vi "Unflatten-EventType.vi"(8 "error in (no error)":errorcluster, 11 "Event Binary Data In":string) -> (0 "error out":errorcluster, 3 "EventType":T1=enum."SDL_EVENT_QUIT")   [LabVIEW 2026, in "SDL3.lvlib" / "Events.lvlib"]
uses:
  Events.lvlib
  EventType--enum.ctl
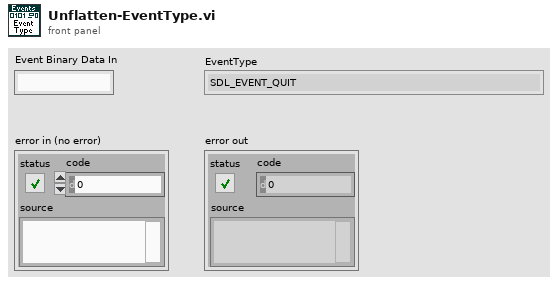
[diagram p1: front panel]
types:
  T1 = typedef "SDL3.lvlib/Events.lvlib/EventType--enum.ctl" = enum16{"LV_NONE", "LV_UNSUPPORTED", "SDL_EVENT_QUIT", "SDL_EVENT_LOCALE_CHANGED", "SDL_EVENT_SYSTEM_THEME_CHANGED", "SDL_EVENT_DISPLAY_ORIENTATION", "SDL_EVENT_DISPLAY_ADDED", "SDL_EVENT_DISPLAY_REMOVED", "SDL_EVENT_DISPLAY_MOVED", "SDL_EVENT_DISPLAY_DESKTOP_MODE_CHANGED", "SDL_EVENT_DISPLAY_CURRENT_MODE_CHANGED", "SDL_EVENT_DISPLAY_CONTENT_SCALE_CHANGED", "SDL_EVENT_WINDOW_SHOWN", "SDL_EVENT_WINDOW_HIDDEN", "SDL_EVENT_WINDOW_EXPOSED", "SDL_EVENT_WINDOW_MOVED", "SDL_EVENT_WINDOW_RESIZED", "SDL_EVENT_WINDOW_PIXEL_SIZE_CHANGED", "SDL_EVENT_WINDOW_METAL_VIEW_RESIZED", "SDL_EVENT_WINDOW_MINIMIZED", "SDL_EVENT_WINDOW_MAXIMIZED", "SDL_EVENT_WINDOW_RESTORED", "SDL_EVENT_WINDOW_MOUSE_ENTER", "SDL_EVENT_WINDOW_MOUSE_LEAVE", "SDL_EVENT_WINDOW_FOCUS_GAINED", "SDL_EVENT_WINDOW_FOCUS_LOST", "SDL_EVENT_WINDOW_CLOSE_REQUESTED", "SDL_EVENT_WINDOW_HIT_TEST", "SDL_EVENT_WINDOW_ICCPROF_CHANGED", "SDL_EVENT_WINDOW_DISPLAY_CHANGED", "SDL_EVENT_WINDOW_DISPLAY_SCALE_CHANGED", "SDL_EVENT_WINDOW_SAFE_AREA_CHANGED", "SDL_EVENT_WINDOW_OCCLUDED", "SDL_EVENT_WINDOW_ENTER_FULLSCREEN", "SDL_EVENT_WINDOW_LEAVE_FULLSCREEN", "SDL_EVENT_WINDOW_DESTROYED", "SDL_EVENT_WINDOW_HDR_STATE_CHANGED", "SDL_EVENT_KEY_DOWN", "SDL_EVENT_KEY_UP", "SDL_EVENT_TEXT_EDITING", "SDL_EVENT_TEXT_INPUT", "SDL_EVENT_KEYMAP_CHANGED", "SDL_EVENT_KEYBOARD_ADDED", "SDL_EVENT_KEYBOARD_REMOVED", "SDL_EVENT_TEXT_EDITING_CANDIDATES", "SDL_EVENT_MOUSE_MOTION", "SDL_EVENT_MOUSE_BUTTON_DOWN", "SDL_EVENT_MOUSE_BUTTON_UP", "SDL_EVENT_MOUSE_WHEEL", "SDL_EVENT_MOUSE_ADDED", "SDL_EVENT_MOUSE_REMOVED", "SDL_EVENT_JOYSTICK_AXIS_MOTION", "SDL_EVENT_JOYSTICK_BALL_MOTION", "SDL_EVENT_JOYSTICK_HAT_MOTION", "SDL_EVENT_JOYSTICK_BUTTON_DOWN", "SDL_EVENT_JOYSTICK_BUTTON_UP", "SDL_EVENT_JOYSTICK_ADDED", "SDL_EVENT_JOYSTICK_REMOVED", "SDL_EVENT_JOYSTICK_BATTERY_UPDATED", "SDL_EVENT_JOYSTICK_UPDATE_COMPLETE", "SDL_EVENT_GAMEPAD_AXIS_MOTION", "SDL_EVENT_GAMEPAD_BUTTON_DOWN", "SDL_EVENT_GAMEPAD_BUTTON_UP", "SDL_EVENT_GAMEPAD_ADDED", "SDL_EVENT_GAMEPAD_REMOVED", "SDL_EVENT_GAMEPAD_REMAPPED", "SDL_EVENT_GAMEPAD_TOUCHPAD_DOWN", "SDL_EVENT_GAMEPAD_TOUCHPAD_MOTION", "SDL_EVENT_GAMEPAD_TOUCHPAD_UP", "SDL_EVENT_GAMEPAD_SENSOR_UPDATE", "SDL_EVENT_GAMEPAD_UPDATE_COMPLETE", "SDL_EVENT_GAMEPAD_STEAM_HANDLE_UPDATED", "SDL_EVENT_FINGER_DOWN", "SDL_EVENT_FINGER_UP", "SDL_EVENT_FINGER_MOTION", "SDL_EVENT_CLIPBOARD_UPDATE", "SDL_EVENT_DROP_FILE", "SDL_EVENT_DROP_TEXT", "SDL_EVENT_DROP_BEGIN", "SDL_EVENT_DROP_COMPLETE", "SDL_EVENT_DROP_POSITION", "SDL_EVENT_AUDIO_DEVICE_ADDED", "SDL_EVENT_AUDIO_DEVICE_REMOVED", "SDL_EVENT_AUDIO_DEVICE_FORMAT_CHANGED", "SDL_EVENT_SENSOR_UPDATE", "SDL_EVENT_PEN_PROXIMITY_IN", "SDL_EVENT_PEN_PROXIMITY_OUT", "SDL_EVENT_PEN_DOWN", "SDL_EVENT_PEN_UP", "SDL_EVENT_PEN_BUTTON_DOWN", "SDL_EVENT_PEN_BUTTON_UP", "SDL_EVENT_PEN_MOTION", "SDL_EVENT_PEN_AXIS", "SDL_EVENT_CAMERA_DEVICE_ADDED", "SDL_EVENT_CAMERA_DEVICE_REMOVED", "SDL_EVENT_CAMERA_DEVICE_APPROVED", "SDL_EVENT_CAMERA_DEVICE_DENIED", "SDL_EVENT_RENDER_TARGETS_RESET", "SDL_EVENT_RENDER_DEVICE_RESET", "SDL_EVENT_POLL_SENTINEL", "SDL_EVENT_USER"}
  T2 = enum16{"big-endian, network order", "native, host order", "little-endian"}
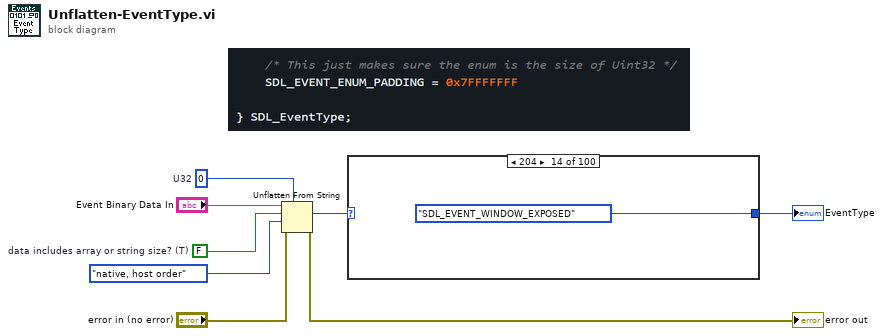
[diagram p0: block diagram]
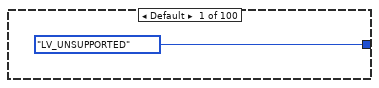
[diagram p2: hidden frame]
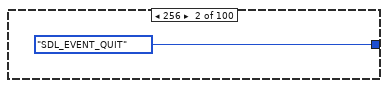
[diagram p3: hidden frame]
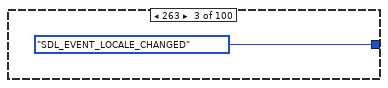
[diagram p4: hidden frame]
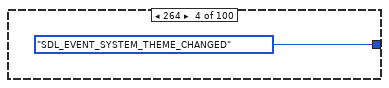
[diagram p5: hidden frame]
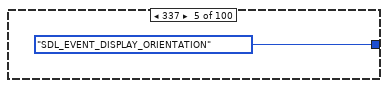
[diagram p6: hidden frame]
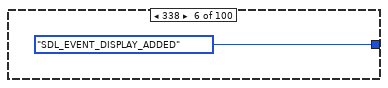
[diagram p7: hidden frame]
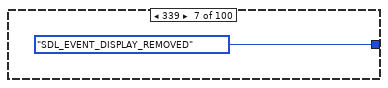
[diagram p8: hidden frame]
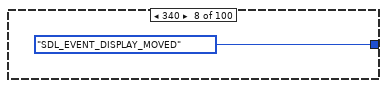
[diagram p9: hidden frame]
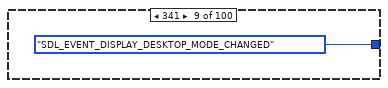
[diagram p10: hidden frame]
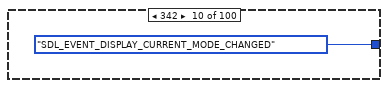
[diagram p11: hidden frame]
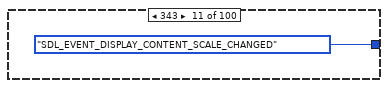
[diagram p12: hidden frame]
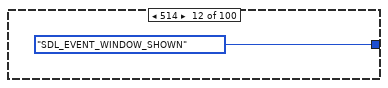
[diagram p13: hidden frame]
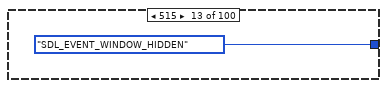
[diagram p14: hidden frame]
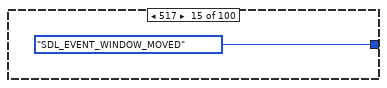
[diagram p15: hidden frame]
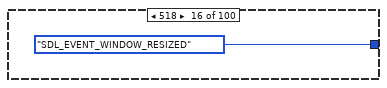
[diagram p16: hidden frame]
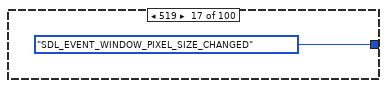
[diagram p17: hidden frame]
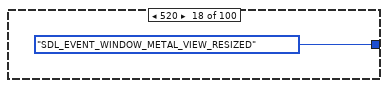
[diagram p18: hidden frame]
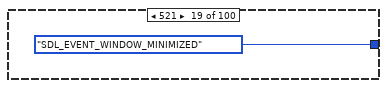
[diagram p19: hidden frame]
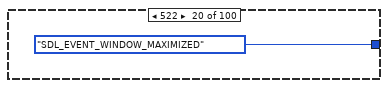
[diagram p20: hidden frame]
diagram:
  w4 = 0  # U32
  w5 = FALSE  # data includes array or string size? (T)
  n1 = Unflatten From String(type=w4, binary string="Event Binary Data In", data includes array or string size? (T)=w5, byte order (0:big-endian, network order)=T2."native, host order", error in (no error)="error in (no error)") -> (value=w2:i32, error out=→"error out":errorcluster)  [unwired: 1 out]
  n2 = case shown="204" w2 {
    tunnel: [EventType--enum."LV_UNSUPPORTED" ("EventType") EventType--enum."SDL_EVENT_QUIT" ("EventType") EventType--enum."SDL_EVENT_LOCALE_CHANGED" ("EventType") EventType--enum."SDL_EVENT_SYSTEM_THEME_CHANGED" ("EventType") EventType--enum."SDL_EVENT_DISPLAY_ORIENTATION" ("EventType") EventType--enum."SDL_EVENT_DISPLAY_ADDED" ("EventType") EventType--enum."SDL_EVENT_DISPLAY_REMOVED" ("EventType") EventType--enum."SDL_EVENT_DISPLAY_MOVED" ("EventType") EventType--enum."SDL_EVENT_DISPLAY_DESKTOP_MODE_CHANGED" ("EventType") EventType--enum."SDL_EVENT_DISPLAY_CURRENT_MODE_CHANGED" ("EventType") EventType--enum."SDL_EVENT_DISPLAY_CONTENT_SCALE_CHANGED" ("EventType") EventType--enum."SDL_EVENT_WINDOW_SHOWN" ("EventType") EventType--enum."SDL_EVENT_WINDOW_HIDDEN" ("EventType") EventType--enum."SDL_EVENT_WINDOW_EXPOSED" ("EventType") EventType--enum."SDL_EVENT_WINDOW_MOVED" ("EventType") EventType--enum."SDL_EVENT_WINDOW_RESIZED" ("EventType") EventType--enum."SDL_EVENT_WINDOW_PIXEL_SIZE_CHANGED" ("EventType") EventType--enum."SDL_EVENT_WINDOW_METAL_VIEW_RESIZED" ("EventType") EventType--enum."SDL_EVENT_WINDOW_MINIMIZED" ("EventType") EventType--enum."SDL_EVENT_WINDOW_MAXIMIZED" ("EventType") EventType--enum."SDL_EVENT_WINDOW_RESTORED" ("EventType") EventType--enum."SDL_EVENT_WINDOW_MOUSE_ENTER" ("EventType") EventType--enum."SDL_EVENT_WINDOW_MOUSE_LEAVE" ("EventType") EventType--enum."SDL_EVENT_WINDOW_FOCUS_GAINED" ("EventType") EventType--enum."SDL_EVENT_WINDOW_FOCUS_LOST" ("EventType") EventType--enum."SDL_EVENT_WINDOW_CLOSE_REQUESTED" ("EventType") EventType--enum."SDL_EVENT_WINDOW_HIT_TEST" ("EventType") EventType--enum."SDL_EVENT_WINDOW_ICCPROF_CHANGED" ("EventType") EventType--enum."SDL_EVENT_WINDOW_DISPLAY_CHANGED" ("EventType") EventType--enum."SDL_EVENT_WINDOW_DISPLAY_SCALE_CHANGED" ("EventType") EventType--enum."SDL_EVENT_WINDOW_SAFE_AREA_CHANGED" ("EventType") EventType--enum."SDL_EVENT_WINDOW_OCCLUDED" ("EventType") EventType--enum."SDL_EVENT_WINDOW_ENTER_FULLSCREEN" ("EventType") EventType--enum."SDL_EVENT_WINDOW_LEAVE_FULLSCREEN" ("EventType") EventType--enum."SDL_EVENT_WINDOW_DESTROYED" ("EventType") EventType--enum."SDL_EVENT_WINDOW_HDR_STATE_CHANGED" ("EventType") EventType--enum."SDL_EVENT_KEY_DOWN" ("EventType") EventType--enum."SDL_EVENT_KEY_UP" ("EventType") EventType--enum."SDL_EVENT_TEXT_EDITING" ("EventType") EventType--enum."SDL_EVENT_TEXT_INPUT" ("EventType") EventType--enum."SDL_EVENT_KEYMAP_CHANGED" ("EventType") EventType--enum."SDL_EVENT_KEYBOARD_ADDED" ("EventType") EventType--enum."SDL_EVENT_KEYBOARD_REMOVED" ("EventType") EventType--enum."SDL_EVENT_TEXT_EDITING_CANDIDATES" ("EventType") EventType--enum."SDL_EVENT_MOUSE_MOTION" ("EventType") EventType--enum."SDL_EVENT_MOUSE_BUTTON_DOWN" ("EventType") EventType--enum."SDL_EVENT_MOUSE_BUTTON_UP" ("EventType") EventType--enum."SDL_EVENT_MOUSE_WHEEL" ("EventType") EventType--enum."SDL_EVENT_MOUSE_ADDED" ("EventType") EventType--enum."SDL_EVENT_MOUSE_REMOVED" ("EventType") EventType--enum."SDL_EVENT_JOYSTICK_AXIS_MOTION" ("EventType") EventType--enum."SDL_EVENT_JOYSTICK_BALL_MOTION" ("EventType") EventType--enum."SDL_EVENT_JOYSTICK_HAT_MOTION" ("EventType") EventType--enum."SDL_EVENT_JOYSTICK_BUTTON_DOWN" ("EventType") EventType--enum."SDL_EVENT_JOYSTICK_BUTTON_UP" ("EventType") EventType--enum."SDL_EVENT_JOYSTICK_ADDED" ("EventType") EventType--enum."SDL_EVENT_JOYSTICK_REMOVED" ("EventType") EventType--enum."SDL_EVENT_JOYSTICK_BATTERY_UPDATED" ("EventType") EventType--enum."SDL_EVENT_JOYSTICK_UPDATE_COMPLETE" ("EventType") EventType--enum."SDL_EVENT_GAMEPAD_AXIS_MOTION" ("EventType") EventType--enum."SDL_EVENT_GAMEPAD_BUTTON_DOWN" ("EventType") EventType--enum."SDL_EVENT_GAMEPAD_BUTTON_UP" ("EventType") EventType--enum."SDL_EVENT_GAMEPAD_ADDED" ("EventType") EventType--enum."SDL_EVENT_GAMEPAD_REMOVED" ("EventType") EventType--enum."SDL_EVENT_GAMEPAD_REMAPPED" ("EventType") EventType--enum."SDL_EVENT_GAMEPAD_TOUCHPAD_DOWN" ("EventType") EventType--enum."SDL_EVENT_GAMEPAD_TOUCHPAD_MOTION" ("EventType") EventType--enum."SDL_EVENT_GAMEPAD_TOUCHPAD_UP" ("EventType") EventType--enum."SDL_EVENT_GAMEPAD_SENSOR_UPDATE" ("EventType") EventType--enum."SDL_EVENT_GAMEPAD_UPDATE_COMPLETE" ("EventType") EventType--enum."SDL_EVENT_GAMEPAD_STEAM_HANDLE_UPDATED" ("EventType") EventType--enum."SDL_EVENT_FINGER_DOWN" ("EventType") EventType--enum."SDL_EVENT_FINGER_UP" ("EventType") EventType--enum."SDL_EVENT_FINGER_MOTION" ("EventType") EventType--enum."SDL_EVENT_CLIPBOARD_UPDATE" ("EventType") EventType--enum."SDL_EVENT_DROP_FILE" ("EventType") EventType--enum."SDL_EVENT_DROP_TEXT" ("EventType") EventType--enum."SDL_EVENT_DROP_BEGIN" ("EventType") EventType--enum."SDL_EVENT_DROP_COMPLETE" ("EventType") EventType--enum."SDL_EVENT_DROP_POSITION" ("EventType") EventType--enum."SDL_EVENT_AUDIO_DEVICE_ADDED" ("EventType") EventType--enum."SDL_EVENT_AUDIO_DEVICE_REMOVED" ("EventType") EventType--enum."SDL_EVENT_AUDIO_DEVICE_FORMAT_CHANGED" ("EventType") EventType--enum."SDL_EVENT_SENSOR_UPDATE" ("EventType") EventType--enum."SDL_EVENT_PEN_PROXIMITY_IN" ("EventType") EventType--enum."SDL_EVENT_PEN_PROXIMITY_OUT" ("EventType") EventType--enum."SDL_EVENT_PEN_DOWN" ("EventType") EventType--enum."SDL_EVENT_PEN_UP" ("EventType") EventType--enum."SDL_EVENT_PEN_BUTTON_DOWN" ("EventType") EventType--enum."SDL_EVENT_PEN_BUTTON_UP" ("EventType") EventType--enum."SDL_EVENT_PEN_MOTION" ("EventType") EventType--enum."SDL_EVENT_PEN_AXIS" ("EventType") EventType--enum."SDL_EVENT_CAMERA_DEVICE_ADDED" ("EventType") EventType--enum."SDL_EVENT_CAMERA_DEVICE_REMOVED" ("EventType") EventType--enum."SDL_EVENT_CAMERA_DEVICE_APPROVED" ("EventType") EventType--enum."SDL_EVENT_CAMERA_DEVICE_DENIED" ("EventType") EventType--enum."SDL_EVENT_RENDER_TARGETS_RESET" ("EventType") EventType--enum."SDL_EVENT_RENDER_DEVICE_RESET" ("EventType") EventType--enum."SDL_EVENT_POLL_SENTINEL" ("EventType") EventType--enum."SDL_EVENT_USER" ("EventType")] -> w1
    frame Default {
    }
    frame 256 {
    }
    frame 263 {
    }
    frame 264 {
    }
    frame 337 {
    }
    frame 338 {
    }
    frame 339 {
    }
    frame 340 {
    }
    frame 341 {
    }
    frame 342 {
    }
    frame 343 {
    }
    frame 514 {
    }
    frame 515 {
    }
    frame 516 {
    }
    frame 517 {
    }
    frame 518 {
    }
    frame 519 {
    }
    frame 520 {
    }
    frame 521 {
    }
    frame 522 {
    }
    frame 523 {
    }
    frame 524 {
    }
    frame 525 {
    }
    frame 526 {
    }
    frame 527 {
    }
    frame 528 {
    }
    frame 529 {
    }
    frame 530 {
    }
    frame 531 {
    }
    frame 532 {
    }
    frame 533 {
    }
    frame 534 {
    }
    frame 535 {
    }
    frame 536 {
    }
    frame 537 {
    }
    frame 538 {
    }
    frame 768 {
    }
    frame 769 {
    }
    frame 770 {
    }
    frame 771 {
    }
    frame 772 {
    }
    frame 773 {
    }
    frame 774 {
    }
    frame 775 {
    }
    frame 1024 {
    }
    frame 1025 {
    }
    frame 1026 {
    }
    frame 1027 {
    }
    frame 1028 {
    }
    frame 1029 {
    }
    frame 1536 {
    }
    frame 1537 {
    }
    frame 1538 {
    }
    frame 1539 {
    }
    frame 1540 {
    }
    frame 1541 {
    }
    frame 1542 {
    }
    frame 1543 {
    }
    frame 1544 {
    }
    frame 1616 {
    }
    frame 1617 {
    }
    frame 1618 {
    }
    frame 1619 {
    }
    frame 1620 {
    }
    frame 1621 {
    }
    frame 1622 {
    }
    frame 1623 {
    }
    frame 1624 {
    }
    frame 1625 {
    }
    frame 1626 {
    }
    frame 1627 {
    }
    frame 1792 {
    }
    frame 1793 {
    }
    frame 1794 {
    }
    frame 2304 {
    }
    frame 4096 {
    }
    frame 4097 {
    }
    frame 4098 {
    }
    frame 4099 {
    }
    frame 4100 {
    }
    frame 4352 {
    }
    frame 4353 {
    }
    frame 4354 {
    }
    frame 4608 {
    }
    frame 4864 {
    }
    frame 4865 {
    }
    frame 4866 {
    }
    frame 4867 {
    }
    frame 4868 {
    }
    frame 4869 {
    }
    frame 4870 {
    }
    frame 4871 {
    }
    frame 5120 {
    }
    frame 5121 {
    }
    frame 5122 {
    }
    frame 5123 {
    }
    frame 8192 {
    }
    frame 8193 {
    }
    frame 32512 {
    }
    frame 32768 {
      # "#ARE_YOU_SURE?"
    }
  }
  "EventType" <- w1
